vi "Function Between Channels.vi"(0 "VISA resource name":refnum<visa-resource-name>, 1 "Function":u16(ring)=204 items=["A1", "A2", "A3", "A4", "A5", "A6", "A7", "A8", "A9", "A10", "A11", "A12", "A13", "A14", "A15", "A16", "A17", "A18", "A19", "A20", "B1", "B2", "B3", "B4", "B5", "B6", "B7", "B8", "B9", "B10", "B11", "B12", "B13", "B14", "B15", "B16", "B17", "B18", "B19", "B20", "C1", "C2", "C3", "C4", "C5", "C6", "C7", "C8", "C9", "C10", "C11", "C12", "C13", "C14", "C15", "C16", "C17", "C18", "C19", "C20", "D1", "D2", "D3", "D4", "D5", "D6", "D7", "D8", "D9", "D10", "D11", "D12", "D13", "D14", "D15", "D16", "D17", "D18", "D19", "D20", "E1", "E2", "E3", "E4", "E5", "E6", "E7", "E8", "E9", "E10", "E11", "E12", "E13", "E14", "E15", "E16", "E17", "E18", "E19", "E20", "F1", "F2", "F3", "F4", "F5", "F6", "F7", "F8", "F9", "F10", "F11", "F12", "F13", "F14", "F15", "F16", "F17", "F18", "F19", "F20", "G1", "G2", "G3", "G4", "G5", "G6", "G7", "G8", "G9", "G10", "G11", "G12", "G13", "G14", "G15", "G16", "G17", "G18", "G19", "G20", "H1", "H2", "H3", "H4", "H5", "H6", "H7", "H8", "H9", "H10", "H11", "H12", "H13", "H14", "H15", "H16", "H17", "H18", "H19", "H20", "I1", "I2", "I3", "I4", "I5", "I6", "I7", "I8", "I9", "I10", "I11", "I12", "I13", "I14", "I15", "I16", "I17", "I18", "I19", "I20", "J1", "J2", "J3", "J4", "J5", "J6", "J7", "J8", "J9", "J10", "J11", "J12", "J13", "J14", "J15", "J16", "J17", "J18", "J19", "J20", "K1", "K2", "K3", "K4", "FA1", "FA2", "FA3", "FA4", "FB1", "FB2", "FB3", "FB4", "FC1", "FC2", "FC3", "FC4", "FD1", "FD2", "FD3", "FD4", "FE1", "FE2", "FE3", "FE4", "FF1", "FF2", "FF3", "FF4", "FG1", "FG2", "FG3", "FG4", "FH1", "FH2", "FH3", "FH4", "FI1", "FI2", "FI3", "FI4", "FJ1", "FJ2", "FJ3", "FJ4"], 2 "Operator":u16(ring) items=["Add", "Substract", "Multiply", "Divide"], 3 "Channel X":u16(ring) items=["A1"=0, "A2"=1, "A3"=2, "A4"=3, "A5"=4, "A6"=5, "A7"=6, "A8"=7, "A9"=8, "A10"=9, "K1"=200, "K2"=201, "K3"=202, "K4"=203, "FA1"=204, "FA2"=205, "FA3"=206, "FA4"=207], 4 "Channel Y":u16(ring) items=["A1"=0, "A2"=1, "A3"=2, "A4"=3, "A5"=4, "A6"=5, "A7"=6, "A8"=7, "A9"=8, "A10"=9, "K1"=200, "K2"=201, "K3"=202, "K4"=203, "FA1"=204, "FA2"=205, "FA3"=206, "FA4"=207], 5 "error in (no error)":errorcluster, 6 "Enable function channel?":bool, 7 "A Coeff.":dbl, 8 "C Coeff.":dbl, 9 "B Coeff.":dbl) -> (14 "VISA resource name out":refnum<visa-resource-name>, 19 "error out":errorcluster)   [LabVIEW 2017, in "Sefram DAS220.lvlib"]
doc: "Function FA1 to FJ4 are used to realize calculations using the following template : aX2+bY+c with X a channel and Y another one.\nYou can also replace the first operator by minus, multiply or divide.\nFor example : a A1^2 - b A5 + c"
uses:
  <instrlib>/Sefram DAS220/Sefram DAS220.lvlib
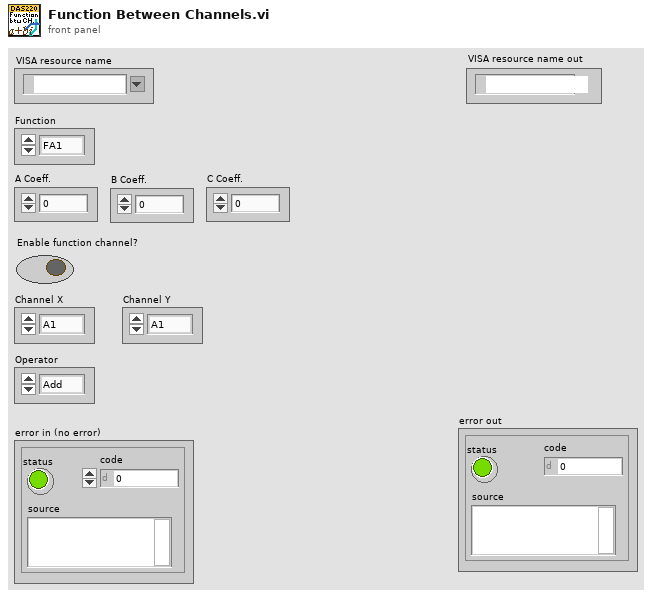
[diagram p1: front panel]
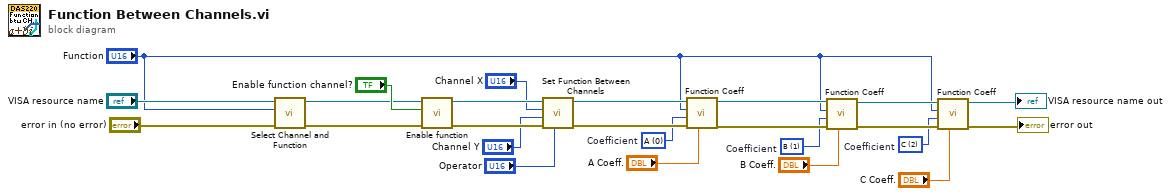
[diagram p0: block diagram]
diagram:
  w8 = u16 2 items=["A", "B", "C", "D", "X1", "X2", "Y1", "Y2"]  # Coefficient
  w9 = u16 1 items=["A", "B", "C", "D", "X1", "X2", "Y1", "Y2"]  # Coefficient
  w10 = u16 0 items=["A", "B", "C", "D", "X1", "X2", "Y1", "Y2"]  # Coefficient
  n1 = call <instrlib>:"Select Channel and Function.vi"("error in (no error)"="error in (no error)", "Channel"="Function", "VISA resource name"="VISA resource name") -> ("error out"=w5:errorcluster, "VISA resource name out"=w6:refnum<visa-resource-name>)  [unwired: 7 in]
  n2 = call <instrlib>:"Enable function.vi"("error in (no error)"=w5, "Enable function channel?"="Enable function channel?", "VISA resource name"=w6) -> ("error out"=w24:errorcluster, "VISA resource name out"=w25:refnum<visa-resource-name>)  [unwired: 7 in]
  n3 = call <instrlib>:"Set Function Between Channels.vi"("Operator"="Operator", "error in (no error)"=w24, "Channel Y"="Channel Y", "Channel X"="Channel X", "VISA resource name"=w25) -> ("error out"=w21:errorcluster, "VISA resource name out"=w22:refnum<visa-resource-name>)  [unwired: 5 in]
  n4 = call <instrlib>:"Function Coeff.vi"("Coefficient value"="A Coeff.", "error in (no error)"=w21, "Coefficient"=w10, "Function"="Function", "VISA resource name"=w22) -> ("error out"=w18:errorcluster, "VISA resource name out"=w19:refnum<visa-resource-name>)  [unwired: 5 in]
  n5 = call <instrlib>:"Function Coeff.vi"("Coefficient value"="B Coeff.", "error in (no error)"=w18, "Coefficient"=w9, "Function"="Function", "VISA resource name"=w19) -> ("error out"=w15:errorcluster, "VISA resource name out"=w16:refnum<visa-resource-name>)  [unwired: 5 in]
  n6 = call <instrlib>:"Function Coeff.vi"("Coefficient value"="C Coeff.", "error in (no error)"=w15, "Coefficient"=w8, "Function"="Function", "VISA resource name"=w16) -> ("error out"=→"error out":errorcluster, "VISA resource name out"=→"VISA resource name out":refnum<visa-resource-name>)  [unwired: 5 in]
